vi "JKI WireTap.vi"(8 "Tap":variant) -> ()   [LabVIEW 2016]
doc: "Worried about alternative data flowing through your wires? Having trouble with a probe that isn't producing any useful information due to an imbalance of power? Order a wiretap! The JKI Wiretap Toolkit uses microwave frequencies to transmit your data wirelessly. Can also be use with IMAQ wires for transmitting camera images."
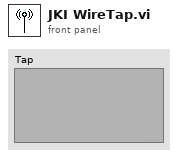
[diagram p1: front panel]
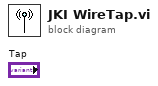
[diagram p0: block diagram]
diagram:
